vi "Ref Curve Optimize Panel.vi"(8 "error in (no error)":errorcluster caption="错误输入（无错误）", 9 "panelHandle":i32, 10 "parentPanelHandle":i32, 11 "asicHandle":i32) -> (0 "error out":errorcluster caption="错误输出", 1 "panelHandle out":i32, 3 "function return":i32)   [LabVIEW 2018]
doc: "extern int __stdcall APSxRefCurveOptimizePanel (int asicHandle, IN int parentPanelHandle, OUT int * panelHandle);"
uses:
  APSx.dll/APSx.dll
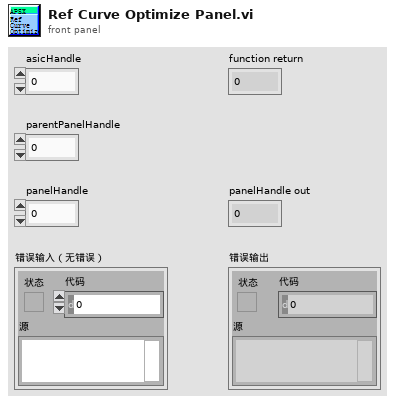
[diagram p1: front panel]
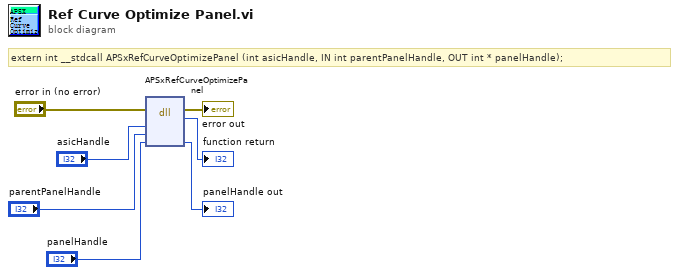
[diagram p0: block diagram]
diagram:
  # "extern int __stdcall APSxRefCurveOptimizePanel (int asicHandle, IN int parentPanelHandle, OUT int * panelHandle);"
  n1 = dll-call lib="PTH2[abs D项目Feng恒隆项目Labview传感器对中台SourcesAPSx.dllAPSx.*" fn="APSxRefCurveOptimizePanel"(error in="error in (no error)", "asicHandle"="asicHandle", "parentPanelHandle"="parentPanelHandle", "panelHandle"="panelHandle") -> (error out=→"error out":errorcluster, →"function return":i32, "panelHandle"=→"panelHandle out":i32)  [unwired: 4 in, 1 out]
